vi "XNET LIN Schedule Entry Property Node.vi"   [LabVIEW 2018]
doc: "Property node used to read/write properties for an XNET LIN Schedule Entry I/O name."
uses:
  <resource>/objmgr/xnet.rc
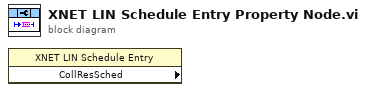
[diagram p0: block diagram]
diagram:
  n1 = property class="XNET LIN Schedule Entry" props=["CollResSched"]() -> ()  [unwired: 2 in, 3 out]
